vi "MathCad15 cmd.vi"(6 "Mathcad15 cmds":T3, 8 "error in":errorcluster, 10 "progress":refnum<vi>, 11 "DesignRequest":T2) -> (0 "first error out":errorcluster, 2 "Mathcad Output":T1, 3 "DesignRequest out":T2)   [LabVIEW 2012, in "Design Server.lvlib"]
uses:
  Design Server.lvlib
  Mathcad15 cmds.ctl
  Design Request.ctl
  Variable cluster.ctl
panel:
  in  "Mathcad.IMathcadApplication":refnum<k7>
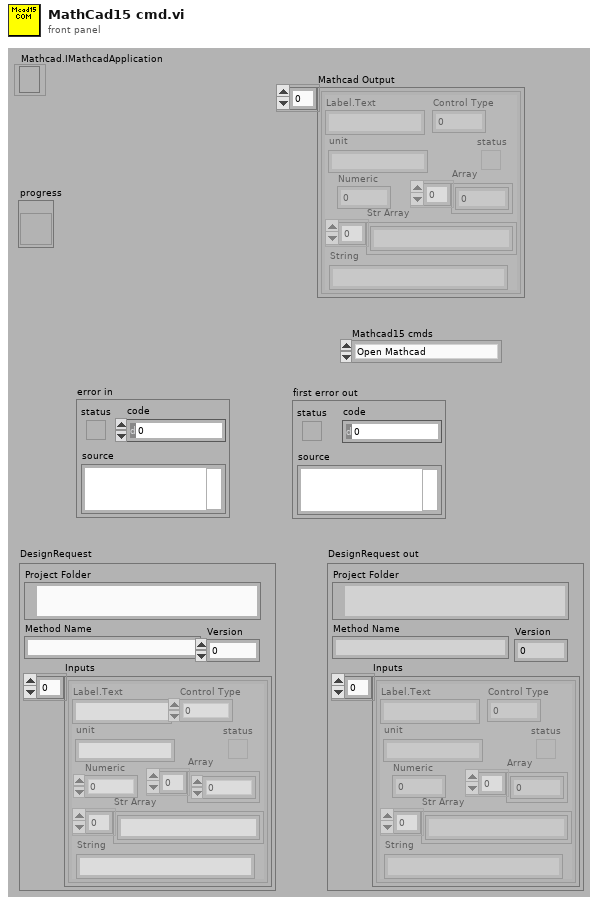
[diagram p1: front panel]
types:
  T1 = typedef "Design Server.lvlib/Variable cluster.ctl" = cluster{"Label.Text":string, "Control Type":u32, "Numeric":dbl, "Array":dbl[], "status":bool, "Str Array":string[], "String":string, "unit":string}[]
  T2 = typedef "Design Server.lvlib/Design Request.ctl" = cluster{"Project Folder":path, "Method Name":string, "Inputs":T1, "Version":i32}
  T3 = typedef "Design Server.lvlib/Mathcad15 cmds.ctl" = enum16{"Open Mathcad", "Execute Method", "Quit Mathcad"}
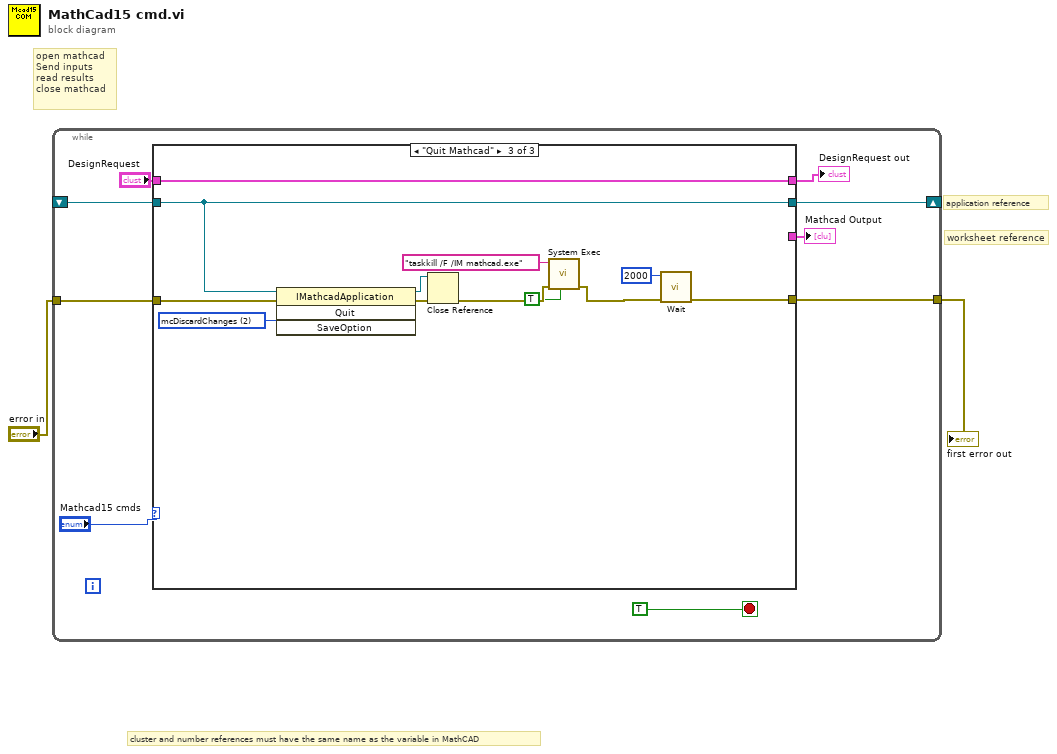
[diagram p0: block diagram]
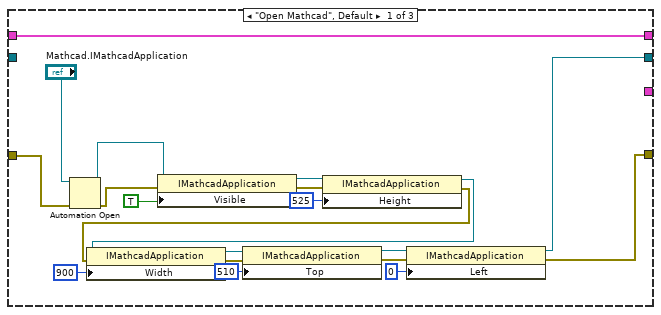
[diagram p2: hidden frame]
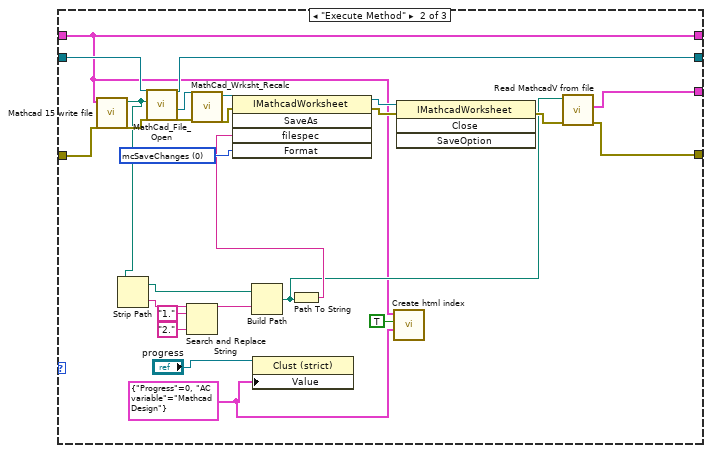
[diagram p3: hidden frame]
diagram:
  # "open mathcad\nSend inputs\nread results\nclose mathcad"
  # "application reference"
  # "worksheet reference"
  # "cluster and number references must have the same name as the variable in MathCAD"
  n1 = while {
    shift-right: [w8] -> _
    shift-left: _ -> [w7]
    tunnel: "error in" -> [w9]
    tunnel: [w10] -> w1
    stop <- TRUE stop-if-true
    n2 = case shown="\"Quit Mathcad\"" "Mathcad15 cmds" {
      tunnel: [w12 w36 w60] -> w10
      tunnel: w9 -> [w29 w57 w64]
      tunnel: [w13 w52 w65] -> w8
      tunnel: w7 -> [_ w53 w65]
      tunnel: [w26 w33 w69] -> w5
      tunnel: "DesignRequest" -> [w26 w33 w69]
      tunnel: [_ w51 _] -> w3
      frame "Open Mathcad", Default {
        n3 = Automation Open(error in (no error)=w29, Automation Refnum="Mathcad.IMathcadApplication") -> (Automation Refnum=w31:refnum<k7>, error out=w30:errorcluster)  [unwired: 2 in]
        n4 = property class="IMathcadApplication"(reference=w31, error in=w30, "Visible"=TRUE) -> (reference out=w24:refnum<k7>, error out=w25:errorcluster)
        n5 = property class="IMathcadApplication"(reference=w24, error in=w25, "Height"=525) -> (reference out=w21:refnum<k7>, error out=w22:errorcluster)
        n6 = property class="IMathcadApplication"(reference=w21, error in=w22, "Width"=900) -> (reference out=w19:refnum<k7>, error out=w18:errorcluster)
        n7 = property class="IMathcadApplication"(reference=w19, error in=w18, "Top"=510) -> (reference out=w16:refnum<k7>, error out=w15:errorcluster)
        n8 = property class="IMathcadApplication"(reference=w16, error in=w15, "Left"=0 ("Top")) -> (reference out=w13:refnum<k7>, error out=w12:errorcluster)
      }
      frame "Execute Method" {
        w32 = cluster{"Progress":u8, "AC variable":string} {"Progress"=0, "AC variable"="Mathcad Design"} ("Value")
        w48 = 0 items=["mcSaveChanges", "mcPromptToSaveChanges", "mcDiscardChanges"] ("SaveOption")
        n9 = call "Mathcad 15 write file.vi"("error in"=w57, "DesignRequest"=w33) -> ("error out"=w56:errorcluster, "Mathcad w inputs"=w38:path)  [unwired: 8 in]
        n10 = Strip Path(path=w38) -> (stripped path=w43:path, name=w47:string)
        n11 = call "MathCad_File_Open.vi"("error in (no error)"=w56, "Worksheet File"=w38, "Mathcad.IMathcadApplication"=w53) -> ("error out (no error)"=w54:errorcluster, "Worksheet Reference"=w55:refnum<k7>, "Application Reference"=w52:refnum<k7>)  [unwired: 5 in, 1 out]
        n12 = Search and Replace String(input string=w47, search string="1.", replace string="2." ("replace string (\"\")")) -> (result string=w44:string)  [unwired: 5 in, 3 out]
        n13 = call "MathCad_Wrksht_Recalc.vi"("error in (no error)"=w54, "Worksheet Reference"=w55) -> ("error out"=w49:errorcluster, "Worksheet Reference"=w50:refnum<k7>)  [unwired: 8 in]
        n14 = Build Path(base path=w43, name or relative path=w44) -> (appended path=w37:path)
        n15 = property class="Clust (strict)"(reference="progress", "Value"=w32) -> ()  [unwired: 1 in, 2 out]
        n16 = Path To String(path=w37) -> (string=w42:string)
        n17 = invoke class="IMathcadWorksheet" method="SaveAs"(reference=w50, error in=w49, "filespec"=w42, "Format"=w48) -> (reference out=w41:refnum<k7>, error out=w40:errorcluster)  [unwired: 1 in, 3 out]
        n18 = call "Create html index.vi"("progress"=w32, "Under construction"=TRUE, "DesignRequest"=w33) -> ()  [unwired: 7 in, 2 out]
        n19 = invoke class="IMathcadWorksheet" method="Close"(reference=w41, error in=w40) -> (error out=w39:errorcluster)  [unwired: 2 in, 3 out]
        n20 = call "Read MathcadV from file.vi"("error in (no error)"=w39, "Path"=w37) -> ("error out"=w36:errorcluster, "Variable Clusters out"=w51:T1)  [unwired: 8 in]
      }
      frame "Quit Mathcad" {
        w66 = 2 items=["mcSaveChanges", "mcPromptToSaveChanges", "mcDiscardChanges"] ("SaveOption")
        n21 = invoke class="IMathcadApplication" method="Quit"(reference=w65, error in=w64, "SaveOption"=w66) -> (reference out=w67:refnum<k7>, error out=w68:errorcluster)  [unwired: 1 in, 2 out]
        n22 = Close Reference(reference=w67, error in (no error)=w68) -> (error out=w62:errorcluster)
        n23 = call <vilib>:"System Exec.vi"("run minimized? (F)"=TRUE, "error in (no error)"=w62, "command line"="taskkill /F /IM mathcad.exe") -> ("error out"=w61:errorcluster)  [unwired: 5 in, 3 out]
        n24 = call "Wait.vi"("error in (no error)"=w61, "milliseconds to wait"=u32 2000) -> ("error out"=w60:errorcluster)  [unwired: 9 in]
      }
    }
    "DesignRequest out" <- w5
    "Mathcad Output" <- w3
  }
  "first error out" <- w1
